vi "MoAgSy_Host_GPG_keyring_p.vi"(0 "MoAgSy_Host":refnum<class "MoAgSy_Host.lvclass">, 2 "key":string, 5 "error in (no error)":errorcluster, 8 "task":T1(ring)) -> (14 "dup MoAgSy_Host":refnum<class "MoAgSy_Host.lvclass">, 16 "pub keys":string[](array[string]), 18 "key":string, 19 "error out":errorcluster)   [LabVIEW 2009, in "MoAgSy.lvlib" / "MoAgSy_Host.lvclass"]
doc: "Use GPG Keyring functions with Hosts GPG object.\nkey input is needed for:\ndelete Key (public key with this id will be removed from hosts keyring)\nadd key (key will be added to keyring)\nlocal sign key (key with this id will be signed by host)\n\nf.berck@gsi.de\nGSI Darmstadt 2009"
uses:
  MoAgSy_Host.lvclass
  MoAgSy_Host.lvclass/MoAgSy_Host.ctl
  MoAgSy_GPG/MoAgSy_GPG.lvclass
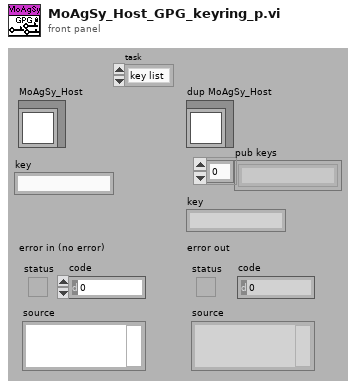
[diagram p1: front panel]
types:
  T1 = enum16{"key list", "pub key", "delete key", "add key", "local sign key"}
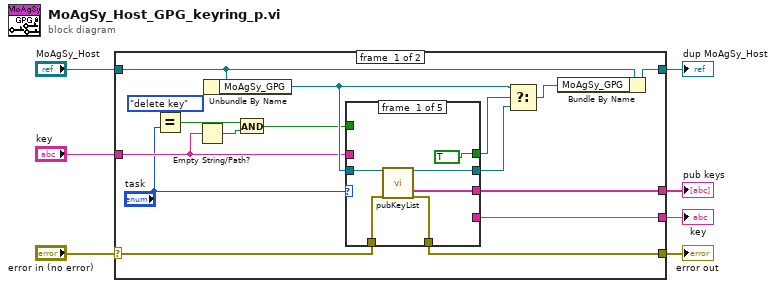
[diagram p0: block diagram]
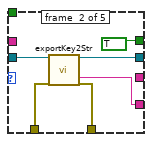
[diagram p2: hidden frame]
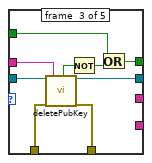
[diagram p3: hidden frame]
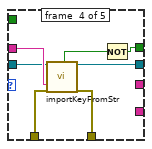
[diagram p4: hidden frame]
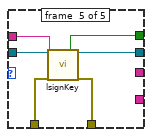
[diagram p5: hidden frame]
diagram:
  n1 = case shown="No Error" "error in (no error)" {
    selector: "error in (no error)" -> [w17 w59]
    tunnel: [w16 w59] -> w6
    tunnel: [w22 w58] -> w4
    tunnel: "MoAgSy_Host" -> [w23 w58]
    tunnel: "key" -> [w12 _]
    tunnel: [w9 _] -> w2
    tunnel: [w8 _] -> w1
    frame #0 {
      n2 = Equal?(x=T1."delete key" ("y"), y="task") -> (x = y?=w14:bool)
      n3 = Empty String/Path?(string/path=w12) -> (empty?=w15:bool)
      n4 = Unbundle By Name(w23) -> ("MoAgSy_GPG"=w21:refnum<class "MoAgSy_GPG.lvclass">)
      n5 = And(x=w14, y=w15) -> (x .and. y?=w11:bool)
      n6 = case shown="\"local sign key\"" "task" {
        tunnel: w21 -> [w29 w35 w44 w48 w57]
        tunnel: [TRUE TRUE w37 w45 w52] -> w18
        tunnel: [w27 w34 w43 w47 w56] -> w19
        tunnel: w17 -> [w26 w32 w42 w50 w54]
        tunnel: [w25 w31 w41 w49 w53] -> w16
        tunnel: [w24 _ _ _ _] -> w9
        tunnel: [_ w30 _ _ _] -> w8
        tunnel: w12 -> [_ _ w40 w51 w55]
        tunnel: w11 -> [_ _ w36 _ _]
        frame #0 {
          n7 = call-dynamic "pubKeyList.vi"("HGF_GPG in"=w29, "error in (no error)"=w26) -> ("HGF_GPG out"=w27:refnum<class "MoAgSy_GPG.lvclass">, "pub keys"=w24:string[], "error out"=w25:errorcluster)  [unwired: 4 in, 11 out]
        }
        frame #1 {
          n8 = call-dynamic "exportKey2Str.vi"("HGF_GPG in"=w35, "error in (no error)"=w32) -> ("HGF_GPG out"=w34:refnum<class "MoAgSy_GPG.lvclass">, "Key"=w30:string, "error out"=w31:errorcluster)  [unwired: 6 in, 9 out]
        }
        frame #2 {
          n9 = call-dynamic "deletePubKey.vi"("HGF_GPG in"=w44, "error in (no error)"=w42, "key-id"=w40) -> ("success"=w39:bool, "HGF_GPG out"=w43:refnum<class "MoAgSy_GPG.lvclass">, "error out"=w41:errorcluster)  [unwired: 4 in, 10 out]
          n10 = Not(x=w39) -> (.not. x?=w38:bool)
          n11 = Or(x=w36, y=w38) -> (x .or. y?=w37:bool)
        }
        frame #3 {
          n12 = call-dynamic "importKeyFromStr.vi"("HGF_GPG in"=w48, "key"=w51, "error in (no error)"=w50) -> ("success"=w46:bool, "HGF_GPG out"=w47:refnum<class "MoAgSy_GPG.lvclass">, "error out"=w49:errorcluster)  [unwired: 4 in, 10 out]
          n13 = Not(x=w46) -> (.not. x?=w45:bool)
        }
        frame #4 {
          n14 = call-dynamic "lsignKey.vi"("MoAgSy_GPG"=w57, "id2sign"=w55, "error in (no error)"=w54) -> ("data error?"=w52:bool, "dup MoAgSy_GPG"=w56:refnum<class "MoAgSy_GPG.lvclass">, "error out"=w53:errorcluster)  [unwired: 6 in, 8 out]
        }
      }
      n15 = Select(t=w21, s=w18, f=w19) -> (s? t:f=w20:refnum<class "MoAgSy_GPG.lvclass">)
      n16 = Bundle By Name(cluster=w23, "MoAgSy_GPG"=w20) -> (w22:refnum<class "MoAgSy_Host.lvclass">)
    }
    frame #1 {
    }
  }
  "error out" <- w6
  "dup MoAgSy_Host" <- w4
  "pub keys" <- w2
  "key" <- w1
